vi "Close Connection.vi"(8 "error in (no error)":errorcluster, 11 "object in":refnum<class "TI.lvclass">) -> (0 "error out":errorcluster, 3 "object out":refnum<class "TI.lvclass">)   [LabVIEW 2020, in "TI.lvclass"]
uses:
  TI.lvclass
  Abstract/Serial Device/Serial Device.lvclass
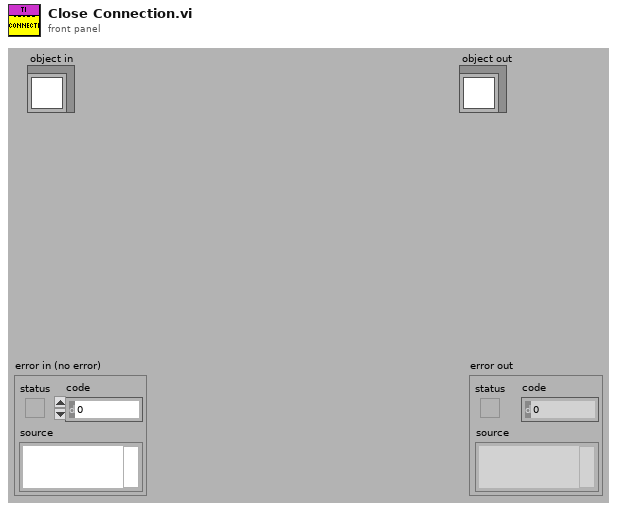
[diagram p1: front panel]
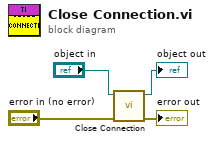
[diagram p0: block diagram]
diagram:
  n1 = call-parent "Close Connection.vi"("error in (no error)"="error in (no error)", "object in"="object in") -> ("error out"=→"error out":errorcluster, "object out"=→"object out":refnum<class "TI.lvclass">)  [unwired: 8 in]
